vi "Test_twosetups_Feb25.vi"() -> ()   [LabVIEW 2015]
uses:
  <vilib>/rvi/Emulation/niFpgaGetClockAttributes.vi
  <vilib>/rvi/Emulation/niFpgaSctlEmulationGetInTimedLoop.vi
  <vilib>/rvi/Emulation/niFpgaEmulationReportErrorSimple.vi
  <vilib>/rvi/eio/common/nirviEmuTemplateMethod_errors.vi
  <vilib>/rvi/interface/RandomDataEmulation/niFpgaRandomDataHandleErrors.vi
  <vilib>/rvi/Emulation/niFpgaCriticalErrorInLSC.vi
  <vilib>/eio/EIONode/EIONode.xnode
  <vilib>/rvi/DataTransferAndStorage/Container/XNode/niFpgaContainer.xnode
  <vilib>/rvi/interface/RandomDataEmulation/nirviRandomDataFpgaReadWriteTemplate.vi
panel:
  out "LED loop time  J8":u32
  out "Loop timer J8":u32
  in  "ConnectorA/AO1 J8":u16
  out "LED loop time J5":u32
  out "loop timer J5":u32
  in  "ConnectorA/AO0 J5":u16
  out "LED loop time J4":u32
  in  "ConnectorB/AO1 J4":u16
  out "Loop time J4":u32
  in  "ConnectorB/AO0 J1":u16
  out "LED loop time":u32
  out "loop timer":u32
  in  "FPGA Stop J4":bool
  out "ConnectorB/DIO0 J4":bool=TRUE
  out "Frame Count J4":i16=5
  in  "IRQ Bit (0-31) J4":u8
  in  "Wait Until IRQ Cleared? J4":bool
  out "Timed Out? J4":bool
  out "ConnectorB/AI0 J4":u16=44020
  out "ConnectorB/DIO1 J4":bool
  in  "double number of samples to take per frame J4":u16=1540
  in  "Half-clocks between frames J4":u16=1600
  in  "stop LED illumination J4":bool
  in  "Low Period (ticks) J4":u32=40000000
  in  "High Period (ticks) J4":u32=40000000
  in  "Apply J4":bool
  out "Tick Count(Ticks) J4":u32 caption="Tick Count(Ticks)"
  in  "Output Enable J4":bool
  in  "FPGA Stop J8":bool
  in  "Half-clock time J8":u32=10
  out "ConnectorA/DIO0 J8":bool=TRUE
  out "Frame Count J8":i16=5
  in  "IRQ Bit (0-31) J8":u8
  in  "Wait Until IRQ Cleared? J8":bool
  out "Timed Out? J8":bool
  out "ConnectorA/AI0 J8":u16=44020
  out "ConnectorA/DIO1 J8":bool
  in  "double number of samples to take per frame J8":u16=1540
  in  "Half-clocks between frames J8":u16=1600
  in  "stop LED illumination J8":bool
  in  "Low Period (ticks) J8":u32=40000000
  in  "High Period (ticks) J8":u32=40000000
  in  "Apply J8":bool
  out "Tick Count(Ticks) J8":u32 caption="Tick Count(Ticks)"
  in  "Output Enable J8":bool
  in  "stop LED illumination J5":bool
  in  "Low Period (ticks) J5":u32=40000000
  in  "High Period (ticks) J5":u32=40000000
  in  "Apply J5":bool
  out "Tick Count(Ticks) J5":u32 caption="Tick Count(Ticks)"
  in  "Output Enable J5":bool
  in  "FPGA Stop J5":bool
  out "ConnectorA/DIO0 J5":bool=TRUE
  out "Frame Count J5":i16=5
  in  "IRQ Bit (0-31) J5":u8
  in  "Wait Until IRQ Cleared? J5":bool
  out "Timed Out? J5":bool
  out "ConnectorA/AI0 J5":u16=44020
  out "ConnectorA/DIO1 J5":bool
  in  "double number of samples to take per frame J5":u16=1540
  in  "Half-clocks between frames J5":u16=1600
  in  "stop LED illumination J1":bool
  in  "Low Period (ticks) J1":u32=40000000
  in  "High Period (ticks) J1":u32=40000000
  in  "Apply J1":bool
  out "Tick Count(Ticks) J1":u32 caption="Tick Count(Ticks)"
  in  "Output Enable J1":bool
  in  "FPGA Stop J1":bool
  out "Frame Count J1":i16=5
  in  "IRQ Bit (0-31) J1":u8
  in  "Wait Until IRQ Cleared? J1":bool
  out "Timed Out? J1":bool
  out "ConnectorB/AI0 J1":u16=44020
  in  "double number of samples to take per frame J1":u16=1540
  in  "Half-clocks between frames J1":u16=1600
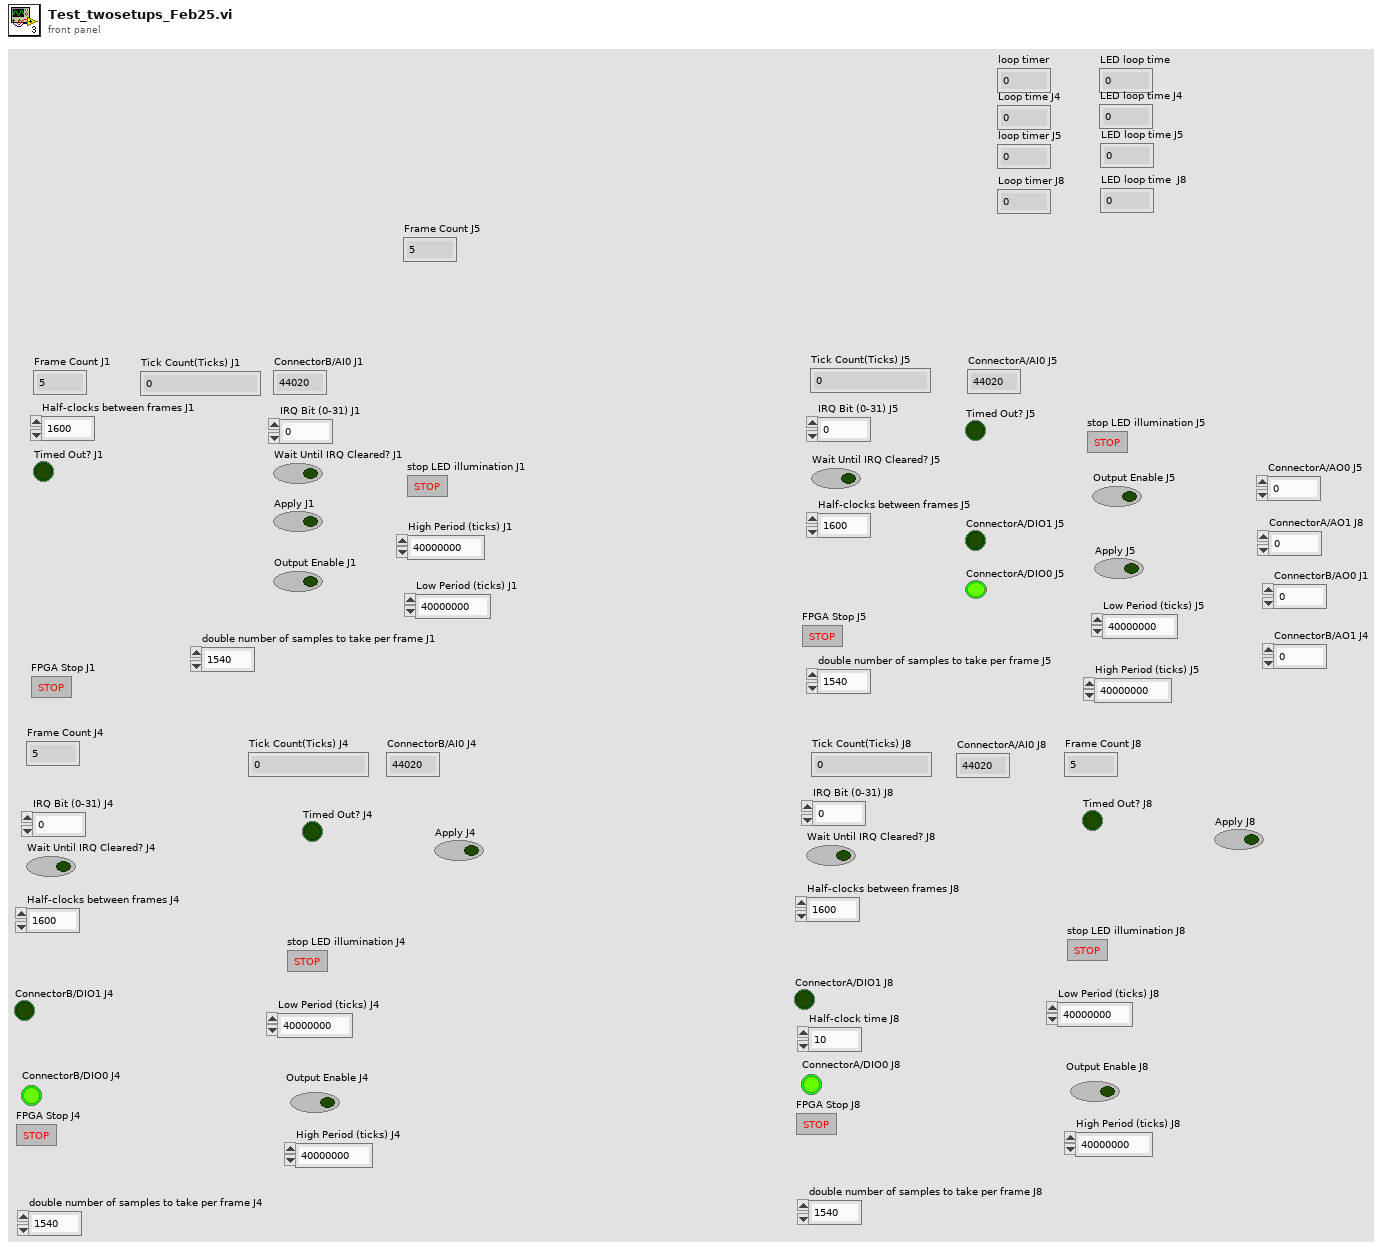
[diagram p1: front panel]
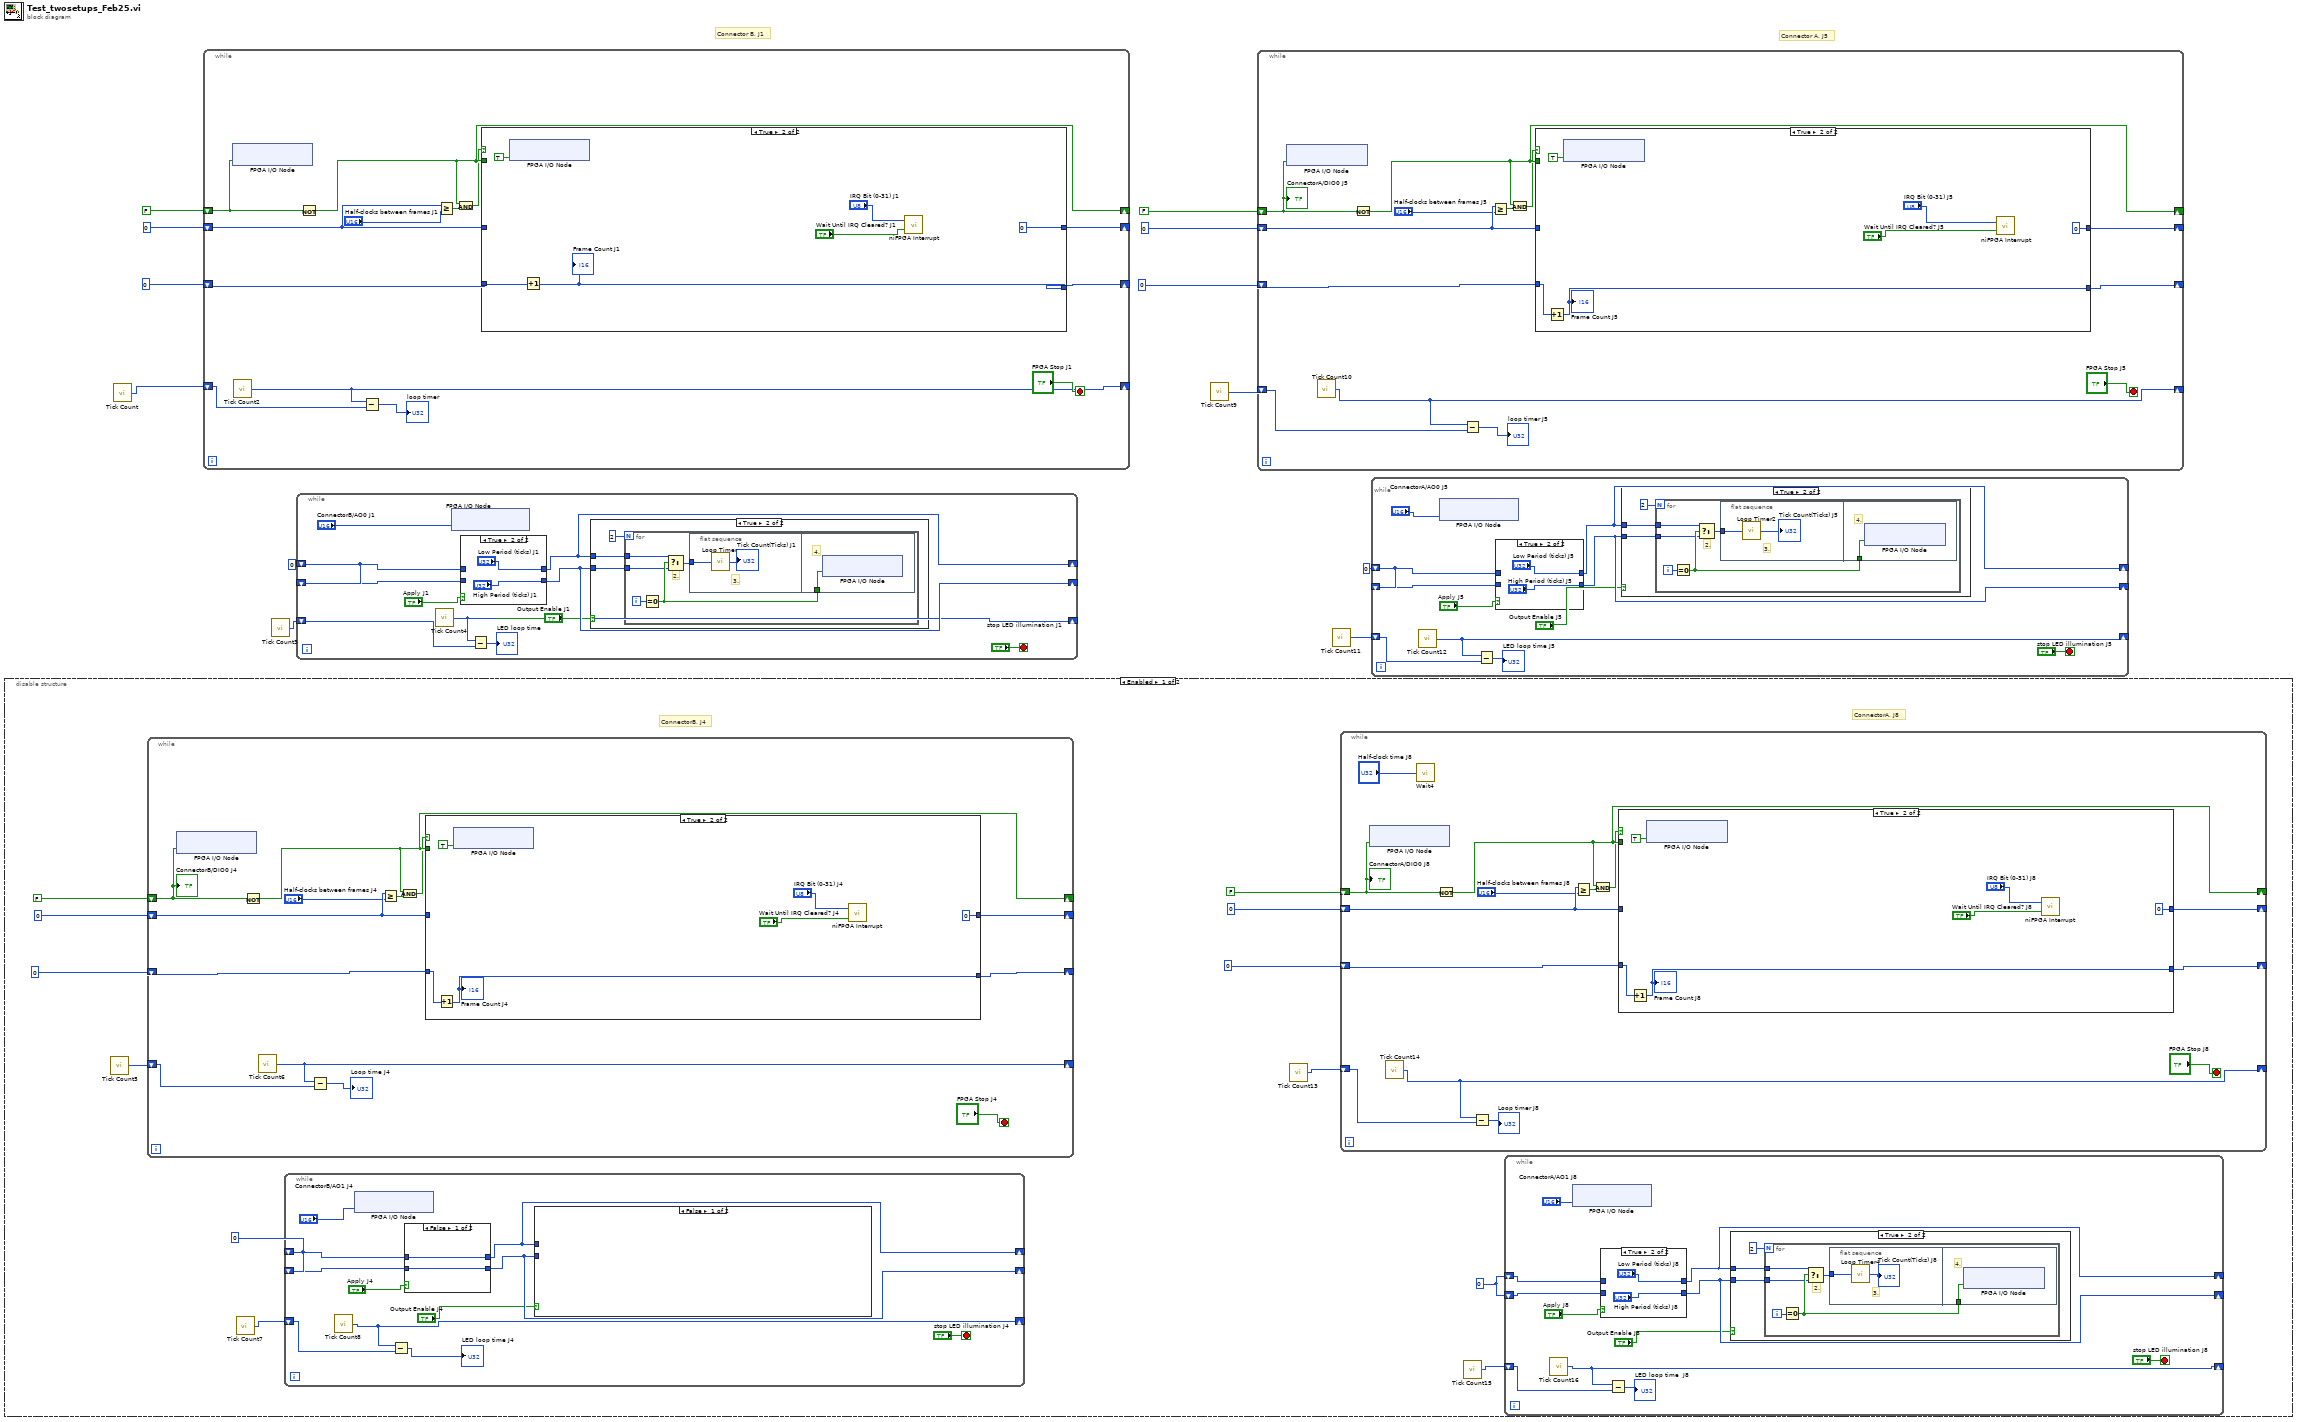
[diagram p0: block diagram]
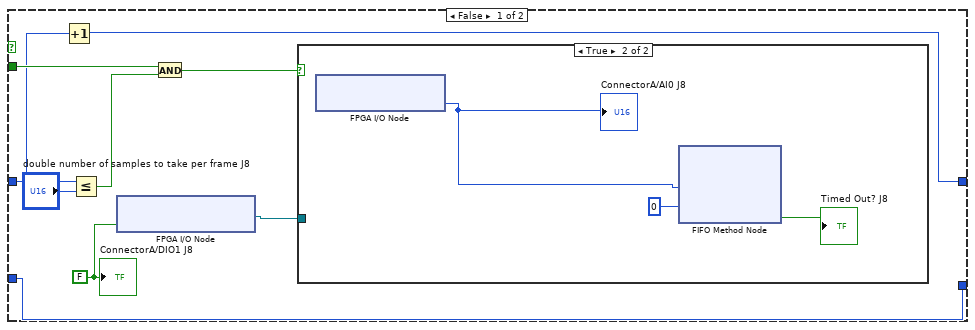
[diagram p4: hidden frame]
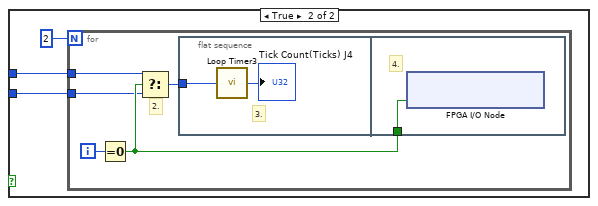
[diagram p6: hidden frame]
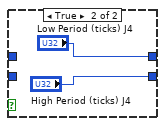
[diagram p7: hidden frame]
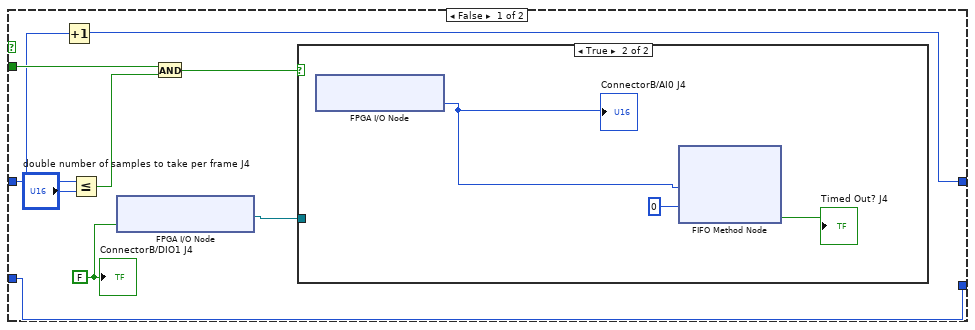
[diagram p8: hidden frame]
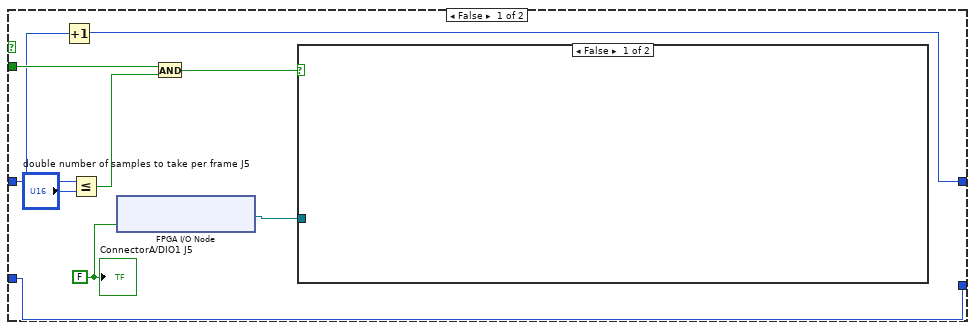
[diagram p13: hidden frame]
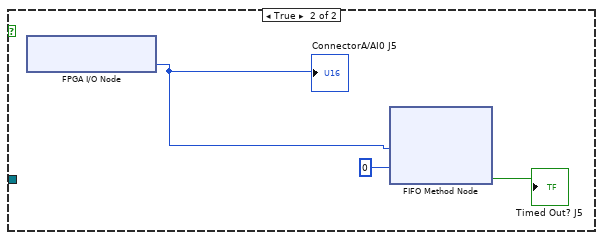
[diagram p14: hidden frame]
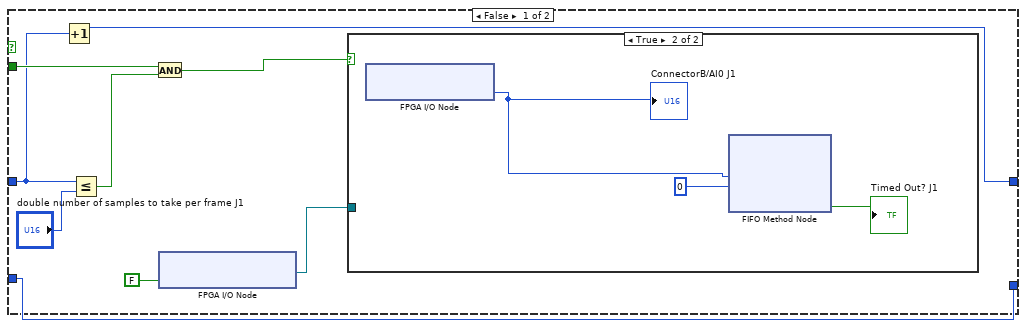
[diagram p17: hidden frame]
diagram:
  w5 = u32 0 ("High Period")
  w9 = u32 0 ("High Period")
  # "Connector A, J5"
  # "Connector B, J1"
  n1 = disable-structure shown="Enabled" {
    frame Enabled {
      w17 = u32 0 ("High Period")
      w21 = u32 0 ("High Period")
      # "ConnectorA, J8"
      # "ConnectorB, J4"
      n2 = call "Tick Count5"() -> ("Tick Count(Ticks)"=w16:u32)
      n3 = while {
        shift-right: [w120] -> _
        shift-left: FALSE ("ConnectorB/DIO0") -> [w121]
        shift-right: [w117] -> _
        shift-left: u16 0 -> [w119]
        shift-right: [w115] -> _
        shift-left: i16 0 -> [w116]
        shift-right: [w111] -> _
        shift-left: w16 -> [w110]
        stop <- "FPGA Stop J4" stop-if-true
        n4 = xnode "FPGA I/O Node"("ConnectorB/DIO2"=w121) -> ()  [unwired: 1 in, 1 out]
        n5 = Not(x=w121) -> (.not. x?=w120:bool)
        n6 = call "Tick Count6"() -> ("Tick Count(Ticks)"=w111:u32)
        n7 = Subtract(x=w111, y=w110) -> (x-y=→"Loop time J4":u32)
        n8 = Greater Or Equal?(x=w119, y="Half-clocks between frames J4") -> (x >= y?=w114:bool)
        n9 = And(x=w120, y=w114) -> (x .and. y?=w112:bool)
        n10 = case shown="True" w112 {
          tunnel: w119 -> [w125 _]
          tunnel: [w123 u16 0] -> w117
          tunnel: w120 -> [w129 _]
          tunnel: w116 -> [w124 w137]
          tunnel: [w124 w136] -> w115
          frame False {
            w130 = FALSE ("ConnectorB/DIO1")
            n11 = Increment(x=w125) -> (x+1=w123:u16)
            n12 = Less Or Equal?(x=w125, y="double number of samples to take per frame J4") -> (x <= y?=w127:bool)
            n13 = xnode "FPGA I/O Node"("ConnectorB/DIO3"=w130) -> ("FPGA I/O Out"=w126:refnum<k21>)  [unwired: 1 in]
            n14 = And(x=w129, y=w127) -> (x .and. y?=w128:bool)
            n15 = case shown="True" w128 {
              tunnel: w126 -> [_ _]
              frame False {
              }
              frame True {
                n16 = xnode "FPGA I/O Node"() -> ("ConnectorB/AI1"=w133:u16)  [unwired: 1 in, 1 out]
                "ConnectorB/AI0 J4" <- w133
                n17 = xnode ("FIFO Method Node")("Element"=w133, "Timeout"=0) -> ("Timed Out?"=→"Timed Out? J4":bool)  [unwired: 1 in, 1 out]
              }
            }
            "ConnectorB/DIO1 J4" <- w130
          }
          frame True {
            n18 = Increment(x=w137) -> (x+1=w136:i16)
            "Frame Count J4" <- w136
            n19 = xnode "FPGA I/O Node"("ConnectorB/DIO3"=TRUE ("ConnectorB/DIO1")) -> ()  [unwired: 1 in, 1 out]
            n20 = call <vilib>:"niFPGA Interrupt.vi"("Wait Until Cleared (F)"="Wait Until IRQ Cleared? J4", "IRQ Number (0)"="IRQ Bit (0-31) J4") -> ()  [unwired: 1 in]
          }
        }
        "ConnectorB/DIO0 J4" <- w121
      }
      n21 = call "Tick Count7"() -> ("Tick Count(Ticks)"=w15:u32)
      n22 = while {
        shift-right: [w88] -> _
        shift-left: w21 -> [w92]
        shift-right: [w89] -> _
        shift-left: w21 -> [w91]
        shift-right: [w85] -> _
        shift-left: w15 -> [w84]
        stop <- "stop LED illumination J4" stop-if-true
        n23 = call "Tick Count8"() -> ("Tick Count(Ticks)"=w85:u32)
        n24 = xnode "FPGA I/O Node"("ConnectorB/AO1"="ConnectorB/AO1 J4") -> ()  [unwired: 1 in, 1 out]
        n25 = Subtract(x=w85, y=w84) -> (x-y=→"LED loop time J4":u32)
        n26 = case shown="False" "Apply J4" {
          tunnel: [w106 "Low Period (ticks) J4"] -> w88
          tunnel: [w105 "High Period (ticks) J4"] -> w89
          tunnel: w92 -> [w106 _]
          tunnel: w91 -> [w105 _]
          frame False {
          }
          frame True {
          }
        }
        n27 = case shown="False" "Output Enable J4" {
          tunnel: w88 -> [_ w95]
          tunnel: w89 -> [_ w94]
          frame False {
          }
          frame True {
            n28 = for {
              N: 2 -> [_]
              tunnel: w95 -> [w98]
              tunnel: w94 -> [w97]
              i -> [w100]
              # "2."
              n29 = Equal To 0?(x=w100) -> (x = 0?=w99:bool)
              n30 = Select(t=w98, s=w99, f=w97) -> (s? t:f=w101:u32)
              n31 = flat-sequence {
                tunnel: w101 -> [w103]
                tunnel: w99 -> [w104]
                frame #0 {
                  # "3."
                  n32 = call "Loop Timer3"("Count(Ticks)"=w103) -> ("Tick Count(Ticks)"=→"Tick Count(Ticks) J4":u32)
                }
                frame #1 {
                  # "4."
                  n33 = xnode "FPGA I/O Node"("ConnectorB/DIO9"=w104) -> ()  [unwired: 1 in, 1 out]
                }
              }
            }
          }
        }
      }
      n34 = call "Tick Count13"() -> ("Tick Count(Ticks)"=w14:u32)
      n35 = while {
        shift-right: [w63] -> _
        shift-left: FALSE ("ConnectorB/DIO0") -> [w64]
        shift-right: [w60] -> _
        shift-left: u16 0 -> [w62]
        shift-right: [w58] -> _
        shift-left: i16 0 -> [w59]
        shift-right: [w52] -> _
        shift-left: w14 -> [w51]
        stop <- "FPGA Stop J8" stop-if-true
        n36 = xnode "FPGA I/O Node"("ConnectorA/DIO2"=w64) -> ()  [unwired: 1 in, 1 out]
        n37 = call "Tick Count14"() -> ("Tick Count(Ticks)"=w52:u32)
        n38 = call "Wait4"("Count(uSec)"="Half-clock time J8") -> ()  [unwired: 1 out]
        n39 = Not(x=w64) -> (.not. x?=w63:bool)
        n40 = Subtract(x=w52, y=w51) -> (x-y=→"Loop timer J8":u32)
        n41 = Greater Or Equal?(x=w62, y="Half-clocks between frames J8") -> (x >= y?=w56:bool)
        n42 = And(x=w63, y=w56) -> (x .and. y?=w54:bool)
        n43 = case shown="True" w54 {
          tunnel: w62 -> [w68 _]
          tunnel: [w66 u16 0] -> w60
          tunnel: w63 -> [w72 _]
          tunnel: w59 -> [w67 w80]
          tunnel: [w67 w79] -> w58
          frame False {
            w73 = FALSE ("ConnectorB/DIO1")
            n44 = Increment(x=w68) -> (x+1=w66:u16)
            n45 = Less Or Equal?(x=w68, y="double number of samples to take per frame J8") -> (x <= y?=w70:bool)
            n46 = xnode "FPGA I/O Node"("ConnectorA/DIO3"=w73) -> ("FPGA I/O Out"=w69:refnum<k21>)  [unwired: 1 in]
            n47 = And(x=w72, y=w70) -> (x .and. y?=w71:bool)
            n48 = case shown="True" w71 {
              tunnel: w69 -> [_ _]
              frame False {
              }
              frame True {
                n49 = xnode "FPGA I/O Node"() -> ("ConnectorA/AI1"=w76:u16)  [unwired: 1 in, 1 out]
                "ConnectorA/AI0 J8" <- w76
                n50 = xnode ("FIFO Method Node")("Element"=w76, "Timeout"=0) -> ("Timed Out?"=→"Timed Out? J8":bool)  [unwired: 1 in, 1 out]
              }
            }
            "ConnectorA/DIO1 J8" <- w73
          }
          frame True {
            n51 = Increment(x=w80) -> (x+1=w79:i16)
            "Frame Count J8" <- w79
            n52 = xnode "FPGA I/O Node"("ConnectorA/DIO3"=TRUE ("ConnectorB/DIO1")) -> ()  [unwired: 1 in, 1 out]
            n53 = call <vilib>:"niFPGA Interrupt.vi"("Wait Until Cleared (F)"="Wait Until IRQ Cleared? J8", "IRQ Number (0)"="IRQ Bit (0-31) J8") -> ()  [unwired: 1 in]
          }
        }
        "ConnectorA/DIO0 J8" <- w64
      }
      n54 = call "Tick Count15"() -> ("Tick Count(Ticks)"=w13:u32)
      n55 = while {
        shift-right: [w30] -> _
        shift-left: w17 -> [w34]
        shift-right: [w31] -> _
        shift-left: w17 -> [w33]
        shift-right: [w25] -> _
        shift-left: w13 -> [w26]
        stop <- "stop LED illumination J8" stop-if-true
        n56 = call "Tick Count16"() -> ("Tick Count(Ticks)"=w25:u32)
        n57 = xnode "FPGA I/O Node"("ConnectorA/AO1"="ConnectorA/AO1 J8") -> ()  [unwired: 1 in, 1 out]
        n58 = case shown="True" "Apply J8" {
          tunnel: [w48 "Low Period (ticks) J8"] -> w30
          tunnel: [w47 "High Period (ticks) J8"] -> w31
          tunnel: w34 -> [w48 _]
          tunnel: w33 -> [w47 _]
          frame False {
          }
          frame True {
          }
        }
        n59 = Subtract(x=w25, y=w26) -> (x-y=→"LED loop time  J8":u32)
        n60 = case shown="True" "Output Enable J8" {
          tunnel: w30 -> [_ w37]
          tunnel: w31 -> [_ w36]
          frame False {
          }
          frame True {
            n61 = for {
              N: 2 -> [_]
              tunnel: w37 -> [w40]
              tunnel: w36 -> [w39]
              i -> [w42]
              # "2."
              n62 = Equal To 0?(x=w42) -> (x = 0?=w41:bool)
              n63 = Select(t=w40, s=w41, f=w39) -> (s? t:f=w43:u32)
              n64 = flat-sequence {
                tunnel: w43 -> [w45]
                tunnel: w41 -> [w46]
                frame #0 {
                  # "3."
                  n65 = call "Loop Timer4"("Count(Ticks)"=w45) -> ("Tick Count(Ticks)"=→"Tick Count(Ticks) J8":u32)
                }
                frame #1 {
                  # "4."
                  n66 = xnode "FPGA I/O Node"("ConnectorA/DIO9"=w46) -> ()  [unwired: 1 in, 1 out]
                }
              }
            }
          }
        }
      }
    }
    frame Disabled {
    }
  }
  n67 = call "Tick Count"() -> ("Tick Count(Ticks)"=w4:u32)
  n68 = while {
    shift-right: [w151] -> _
    shift-left: FALSE ("ConnectorB/DIO0") -> [w152]
    shift-right: [w148] -> _
    shift-left: u16 0 -> [w150]
    shift-right: [w146] -> _
    shift-left: i16 0 -> [w147]
    shift-right: [w142] -> _
    shift-left: w4 -> [w141]
    stop <- "FPGA Stop J1" stop-if-true
    n69 = xnode "FPGA I/O Node"("ConnectorB/DIO0"=w152) -> ()  [unwired: 1 in, 1 out]
    n70 = call "Tick Count2"() -> ("Tick Count(Ticks)"=w142:u32)
    n71 = Not(x=w152) -> (.not. x?=w151:bool)
    n72 = Subtract(x=w142, y=w141) -> (x-y=→"loop timer":u32)
    n73 = Greater Or Equal?(x=w150, y="Half-clocks between frames J1") -> (x >= y?=w145:bool)
    n74 = And(x=w151, y=w145) -> (x .and. y?=w143:bool)
    n75 = case shown="True" w143 {
      tunnel: w150 -> [w156 _]
      tunnel: [w154 u16 0] -> w148
      tunnel: w151 -> [w160 _]
      tunnel: w147 -> [w155 w168]
      tunnel: [w155 w167] -> w146
      frame False {
        n76 = Increment(x=w156) -> (x+1=w154:u16)
        n77 = Less Or Equal?(x=w156, y="double number of samples to take per frame J1") -> (x <= y?=w158:bool)
        n78 = And(x=w160, y=w158) -> (x .and. y?=w159:bool)
        n79 = xnode "FPGA I/O Node"("ConnectorB/DIO1"=FALSE) -> ("FPGA I/O Out"=w157:refnum<k21>)  [unwired: 1 in]
        n80 = case shown="True" w159 {
          tunnel: w157 -> [_ _]
          frame False {
          }
          frame True {
            n81 = xnode "FPGA I/O Node"() -> ("ConnectorB/AI0"=w164:u16)  [unwired: 1 in, 1 out]
            "ConnectorB/AI0 J1" <- w164
            n82 = xnode ("FIFO Method Node")("Element"=w164, "Timeout"=0) -> ("Timed Out?"=→"Timed Out? J1":bool)  [unwired: 1 in, 1 out]
          }
        }
      }
      frame True {
        n83 = xnode "FPGA I/O Node"("ConnectorB/DIO1"=TRUE) -> ()  [unwired: 1 in, 1 out]
        n84 = Increment(x=w168) -> (x+1=w167:i16)
        "Frame Count J1" <- w167
        n85 = call <vilib>:"niFPGA Interrupt.vi"("Wait Until Cleared (F)"="Wait Until IRQ Cleared? J1", "IRQ Number (0)"="IRQ Bit (0-31) J1") -> ()  [unwired: 1 in]
      }
    }
  }
  n86 = call "Tick Count3"() -> ("Tick Count(Ticks)"=w3:u32)
  n87 = while {
    shift-right: [w176] -> _
    shift-left: w9 -> [w180]
    shift-right: [w177] -> _
    shift-left: w9 -> [w179]
    shift-right: [w174] -> _
    shift-left: w3 -> [w173]
    stop <- "stop LED illumination J1" stop-if-true
    n88 = call "Tick Count4"() -> ("Tick Count(Ticks)"=w174:u32)
    n89 = xnode "FPGA I/O Node"("ConnectorB/AO0"="ConnectorB/AO0 J1") -> ()  [unwired: 1 in, 1 out]
    n90 = case shown="True" "Apply J1" {
      tunnel: [w194 "Low Period (ticks) J1"] -> w176
      tunnel: [w193 "High Period (ticks) J1"] -> w177
      tunnel: w180 -> [w194 _]
      tunnel: w179 -> [w193 _]
      frame False {
      }
      frame True {
      }
    }
    n91 = Subtract(x=w174, y=w173) -> (x-y=→"LED loop time":u32)
    n92 = case shown="True" "Output Enable J1" {
      tunnel: w176 -> [_ w183]
      tunnel: w177 -> [_ w182]
      frame False {
      }
      frame True {
        n93 = for {
          N: 2 -> [_]
          tunnel: w183 -> [w186]
          tunnel: w182 -> [w185]
          i -> [w188]
          # "2."
          n94 = Equal To 0?(x=w188) -> (x = 0?=w187:bool)
          n95 = Select(t=w186, s=w187, f=w185) -> (s? t:f=w189:u32)
          n96 = flat-sequence {
            tunnel: w189 -> [w191]
            tunnel: w187 -> [w192]
            frame #0 {
              # "3."
              n97 = call "Loop Timer"("Count(Ticks)"=w191) -> ("Tick Count(Ticks)"=→"Tick Count(Ticks) J1":u32)
            }
            frame #1 {
              # "4."
              n98 = xnode "FPGA I/O Node"("ConnectorB/DIO8"=w192) -> ()  [unwired: 1 in, 1 out]
            }
          }
        }
      }
    }
  }
  n99 = call "Tick Count9"() -> ("Tick Count(Ticks)"=w2:u32)
  n100 = while {
    shift-right: [w208] -> _
    shift-left: FALSE ("ConnectorB/DIO0") -> [w209]
    shift-right: [w205] -> _
    shift-left: u16 0 -> [w207]
    shift-right: [w203] -> _
    shift-left: i16 0 -> [w204]
    shift-right: [w198] -> _
    shift-left: w2 -> [w197]
    stop <- "FPGA Stop J5" stop-if-true
    n101 = xnode "FPGA I/O Node"("ConnectorA/DIO0"=w209) -> ()  [unwired: 1 in, 1 out]
    n102 = call "Tick Count10"() -> ("Tick Count(Ticks)"=w198:u32)
    n103 = Not(x=w209) -> (.not. x?=w208:bool)
    n104 = Subtract(x=w198, y=w197) -> (x-y=→"loop timer J5":u32)
    n105 = Greater Or Equal?(x=w207, y="Half-clocks between frames J5") -> (x >= y?=w202:bool)
    n106 = And(x=w208, y=w202) -> (x .and. y?=w200:bool)
    n107 = case shown="True" w200 {
      tunnel: w207 -> [w213 _]
      tunnel: [w211 u16 0] -> w205
      tunnel: w208 -> [w217 _]
      tunnel: w204 -> [w212 w225]
      tunnel: [w212 w224] -> w203
      frame False {
        w218 = FALSE ("ConnectorB/DIO1")
        n108 = Increment(x=w213) -> (x+1=w211:u16)
        n109 = Less Or Equal?(x=w213, y="double number of samples to take per frame J5") -> (x <= y?=w215:bool)
        n110 = xnode "FPGA I/O Node"("ConnectorA/DIO1"=w218) -> ("FPGA I/O Out"=w214:refnum<k21>)  [unwired: 1 in]
        n111 = And(x=w217, y=w215) -> (x .and. y?=w216:bool)
        n112 = case shown="False" w216 {
          tunnel: w214 -> [_ _]
          frame False {
          }
          frame True {
            n113 = xnode "FPGA I/O Node"() -> ("ConnectorA/AI0"=w221:u16)  [unwired: 1 in, 1 out]
            "ConnectorA/AI0 J5" <- w221
            n114 = xnode ("FIFO Method Node")("Element"=w221, "Timeout"=0) -> ("Timed Out?"=→"Timed Out? J5":bool)  [unwired: 1 in, 1 out]
          }
        }
        "ConnectorA/DIO1 J5" <- w218
      }
      frame True {
        n115 = Increment(x=w225) -> (x+1=w224:i16)
        "Frame Count J5" <- w224
        n116 = xnode "FPGA I/O Node"("ConnectorA/DIO1"=TRUE ("ConnectorB/DIO1")) -> ()  [unwired: 1 in, 1 out]
        n117 = call <vilib>:"niFPGA Interrupt.vi"("Wait Until Cleared (F)"="Wait Until IRQ Cleared? J5", "IRQ Number (0)"="IRQ Bit (0-31) J5") -> ()  [unwired: 1 in]
      }
    }
    "ConnectorA/DIO0 J5" <- w209
  }
  n118 = call "Tick Count11"() -> ("Tick Count(Ticks)"=w1:u32)
  n119 = while {
    shift-right: [w233] -> _
    shift-left: w5 -> [w237]
    shift-right: [w234] -> _
    shift-left: w5 -> [w236]
    shift-right: [w229] -> _
    shift-left: w1 -> [w228]
    stop <- "stop LED illumination J5" stop-if-true
    n120 = call "Tick Count12"() -> ("Tick Count(Ticks)"=w229:u32)
    n121 = xnode "FPGA I/O Node"("ConnectorA/AO0"="ConnectorA/AO0 J5") -> ()  [unwired: 1 in, 1 out]
    n122 = Subtract(x=w229, y=w228) -> (x-y=→"LED loop time J5":u32)
    n123 = case shown="True" "Apply J5" {
      tunnel: [w251 "Low Period (ticks) J5"] -> w233
      tunnel: [w250 "High Period (ticks) J5"] -> w234
      tunnel: w237 -> [w251 _]
      tunnel: w236 -> [w250 _]
      frame False {
      }
      frame True {
      }
    }
    n124 = case shown="True" "Output Enable J5" {
      tunnel: w233 -> [_ w240]
      tunnel: w234 -> [_ w239]
      frame False {
      }
      frame True {
        n125 = for {
          N: 2 -> [_]
          tunnel: w240 -> [w243]
          tunnel: w239 -> [w242]
          i -> [w245]
          # "2."
          n126 = Equal To 0?(x=w245) -> (x = 0?=w244:bool)
          n127 = Select(t=w243, s=w244, f=w242) -> (s? t:f=w246:u32)
          n128 = flat-sequence {
            tunnel: w246 -> [w248]
            tunnel: w244 -> [w249]
            frame #0 {
              # "3."
              n129 = call "Loop Timer2"("Count(Ticks)"=w248) -> ("Tick Count(Ticks)"=→"Tick Count(Ticks) J5":u32)
            }
            frame #1 {
              # "4."
              n130 = xnode "FPGA I/O Node"("ConnectorA/DIO8"=w249) -> ()  [unwired: 1 in, 1 out]
            }
          }
        }
      }
    }
  }
